vi "Filter FGV.vi"(8 "error in (no error)":errorcluster, 10 "GUIDs to Add":string[](array[string]), 11 "Enum":enum16{"Get Filter", "Add GUIDs"}(ring)) -> (0 "error out":errorcluster, 3 "Filter Out":refnum<k24>)   [LabVIEW 2015]
uses:
  NationalInstruments.VeriStand.SystemStorage
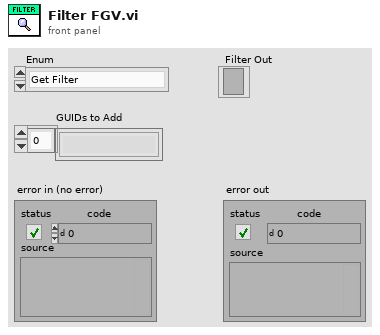
[diagram p1: front panel]
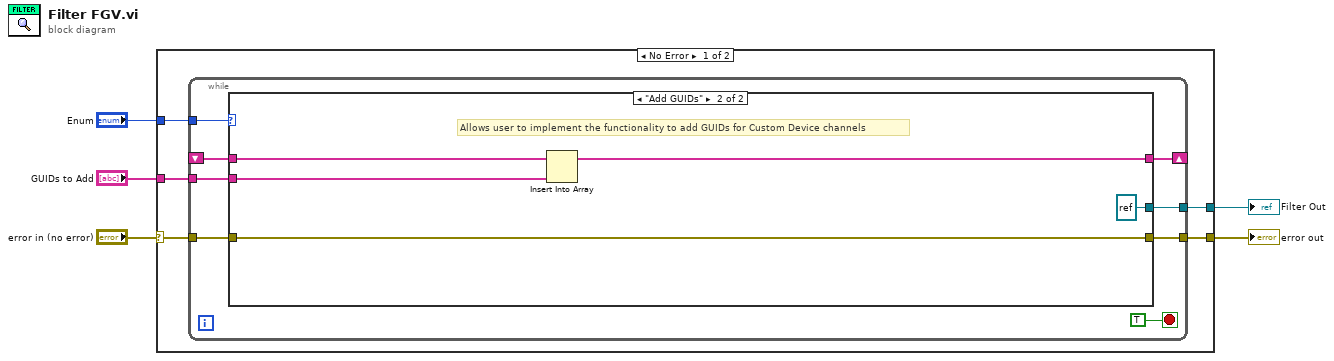
[diagram p0: block diagram]
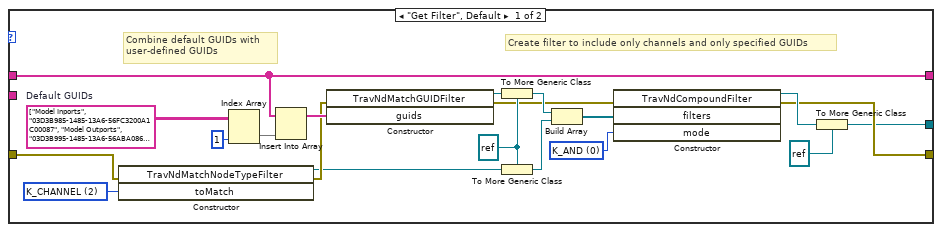
[diagram p2: hidden frame]
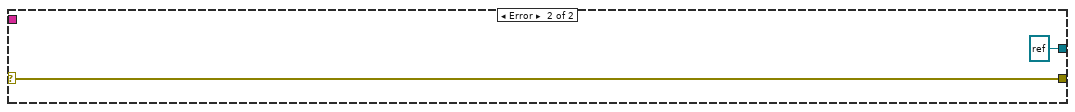
[diagram p3: hidden frame]
diagram:
  n1 = case shown="No Error" "error in (no error)" {
    selector: "error in (no error)" -> [w9 w44]
    tunnel: "GUIDs to Add" -> [w8 _]
    tunnel: "Enum" -> [w10 _]
    tunnel: [w7 w44] -> w2
    tunnel: [w6 refnum<k24> refnum ("customFilter")] -> w1
    frame No Error {
      n2 = while {
        shift-right: [w14] -> _
        shift-left: _ -> [w13]
        tunnel: w10 -> [w17]
        tunnel: w9 -> [w16]
        tunnel: w8 -> [w15]
        tunnel: [w12] -> w7
        tunnel: [w11] -> w6
        stop <- TRUE stop-if-true
        n3 = case shown="\"Add GUIDs\"" w17 {
          tunnel: w16 -> [w32 w40]
          tunnel: w15 -> [_ w43]
          tunnel: [w35 w42] -> w14
          tunnel: w13 -> [w35 w41]
          tunnel: [w20 w40] -> w12
          tunnel: [w19 refnum<k24> refnum ("customFilter")] -> w11
          frame "Get Filter", Default {
            w23 = 0 items=["K_AND", "K_OR"] ("mode")
            w28 = refnum<k24> refnum ("customFilter")
            w33 = 2 items=["K_BASE", "K_ALIAS", "K_CHANNEL", "K_SECTION", "K_TARGET", "K_TARGETSECTION", "K_ROOT", "K_WAVEFORM"] ("toMatch")
            w38 = string[][] [["Model Inports", "03D3B985-1485-13A6-56FC3200A1C00087"], ["Model Outports", "03D3B995-1485-13A6-56ABA0860ADF91DF"], ["AI Channels", "775506CE-1485-13A6-56A13E7139081FC2"], ["AO Channels", "775506DD-1485-13A6-569AA9AEB5FBC117"], ["DI Channels", "775506ED-1485-13A6-56B51E84EB822783"], ["DO Channels", "775506FD-1485-13A6-56399B676D4C3FBE"], ["CI Channels", "7755070C-1485-13A6-56E9A76A19C3486D"], ["CO Frequency", "D0E0AD4A-0211-11E2-9E7C-F95C6188709B"], ["CO Duty Cycle", "C988A160-0211-11E2-8F86-F85C6188709B"], ["FPGA AI", "5F92BE66-C305-11DD-B8A3-E45255D89593"], ["FPGA DI", "CFB42AC2-C305-11DD-A2CF-045755D89593"], ["FPGA PWM In", "EB58352A-C305-11DD-B8C7-165855D89593"], ["FPGA AO", "9A756434-C305-11DD-8CF1-675555D89593"], ["FPGA DO", "DF397312-C305-11DD-9AEF-AD5755D89593"], ["FPGA PWM Out", "FFB4F0E4-C305-11DD-96D3-EA5855D89593"], ["XNET Frames", "7219d3d0-e11d-11de-8a39-0800200c9a66"], ["CD Channel", "03D3BB99-1485-13A6-561D1F898F032919"], ["User Channel", "03D3B6C6-1485-13A6-56609EA3AE19E356"]]  # Default GUIDs
            # "Create filter to include only channels and only specified GUIDs"
            # "Combine default GUIDs with\nuser-defined GUIDs"
            n4 = constructor class="TravNdMatchNodeTypeFilter"(error in=w32, "toMatch"=w33) -> (reference out=w27:refnum<k24>, error out=w31:errorcluster)  [unwired: 2 in, 2 out]
            n5 = Index Array(array=w38, index (col)=1 ("disabled index (col)")) -> (element=w36:string[])  [unwired: 1 in]
            n6 = Insert Into Array(array=w35, new element=w36) -> (w34:string[])  [unwired: 1 in]
            n7 = constructor class="TravNdMatchGUIDFilter"(error in=w31, "guids"=w34) -> (reference out=w30:refnum<k24>, error out=w24:errorcluster)  [unwired: 2 in, 2 out]
            n8 = To More Generic Class(target class=w28, reference=w30) -> (generic class reference=w29:refnum<k24>)
            n9 = To More Generic Class(target class=w28, reference=w27) -> (generic class reference=w26:refnum<k24>)
            n10 = Build Array(w29, w26) -> (w25:refnum<k24>[])
            n11 = constructor class="TravNdCompoundFilter"(error in=w24, "filters"=w25, "mode"=w23) -> (reference out=w21:refnum<k24>, error out=w20:errorcluster)  [unwired: 2 in, 3 out]
            n12 = To More Generic Class(target class=refnum<k24> refnum ("customFilter"), reference=w21) -> (generic class reference=w19:refnum<k24>)
          }
          frame "Add GUIDs" {
            # "Allows user to implement the functionality to add GUIDs for Custom Device channels"
            n13 = Insert Into Array(array=w41, new element=w43) -> (w42:string[])  [unwired: 1 in]
          }
        }
      }
    }
    frame Error {
    }
  }
  "error out" <- w2
  "Filter Out" <- w1
